vi "Filmetrics.vi"() -> ()   [LabVIEW 2018]
uses:
  <vilib>/Utility/file.llb/Write Delimited Spreadsheet (DBL).vi
  <vilib>/Utility/file.llb/Read Delimited Spreadsheet (DBL).vi
panel:
  in  "Accumulation times":sgl=1.0 min=1 step=1 format="%#_1g"
  in  "Substrate":string(combo)
  in  "Accumulation?":bool
  in  "Guessing Thickness(nm)3":string
  in  "Guessing Thickness(nm)2":string
  in  "Guessing Thickness(nm)1":string
  in  "Layer 3 Material":string(combo)
  in  "Layer 2 Material":string(combo)
  in  "Layer 1 Material":string(combo)
  in  "Calculate Thickness":bool
  out "Layers Ready":bool
  in  "Set layers":bool
  in  "Number of layers":sgl=1.0 min=1 max=3 step=1
  out "Raw Intensity Graph":T1(graph)
  out "Reflectance vs. Wavelength Graph":cluster{"all rows":dbl[], "all rows":dbl[]}[](graph)
  out "Display":string
  out "Scan Completed?":bool
  out "Counts":i32
  in  "Measurement":enum16{"Background", "Silicon", "Sample"}(ring)
  in  "Start Scan":bool
  in  "Stop Scan":bool
  in  "Integration Time [s] (0.001)":dbl=0.01 min=0.01
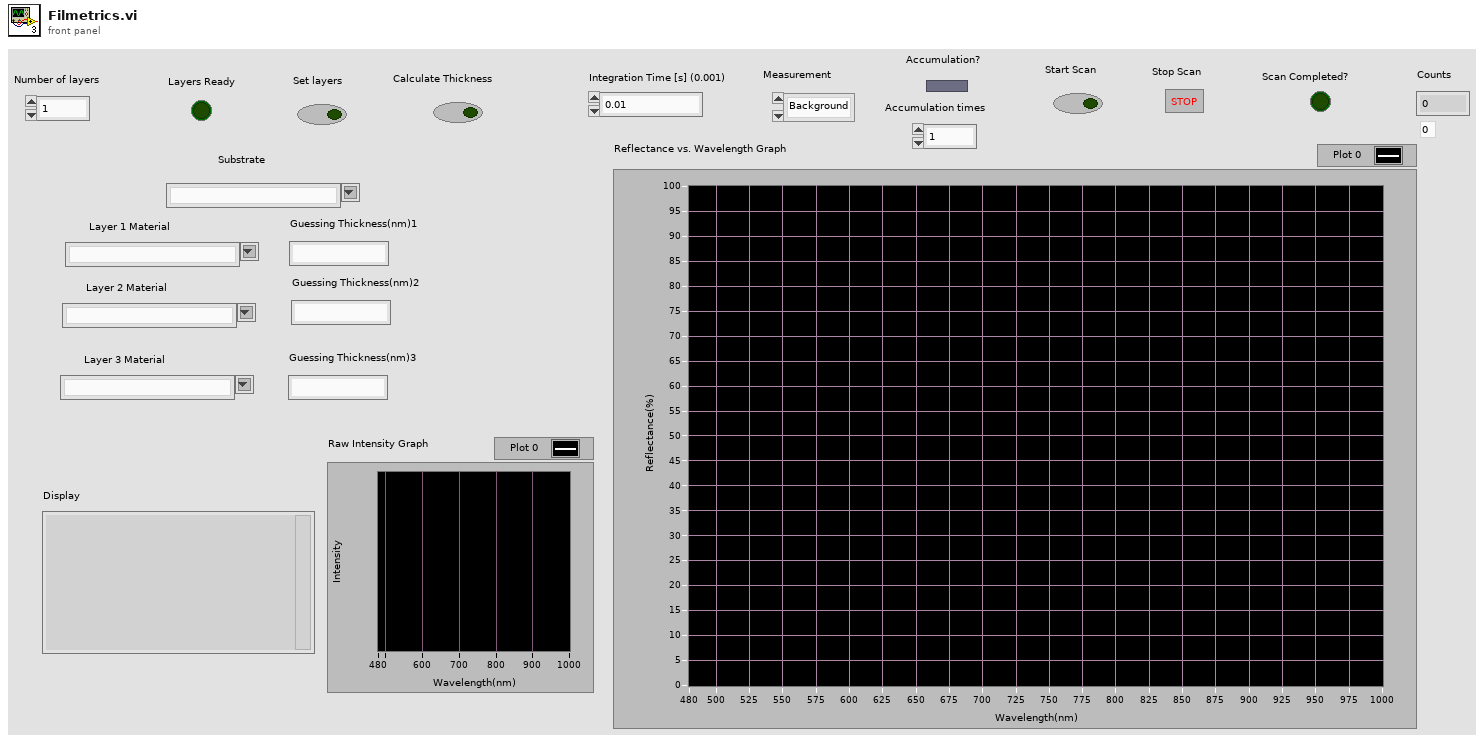
[diagram p1: front panel]
types:
  T1 = cluster{"Wavelength Data Array":dbl[], "Data":dbl[]}
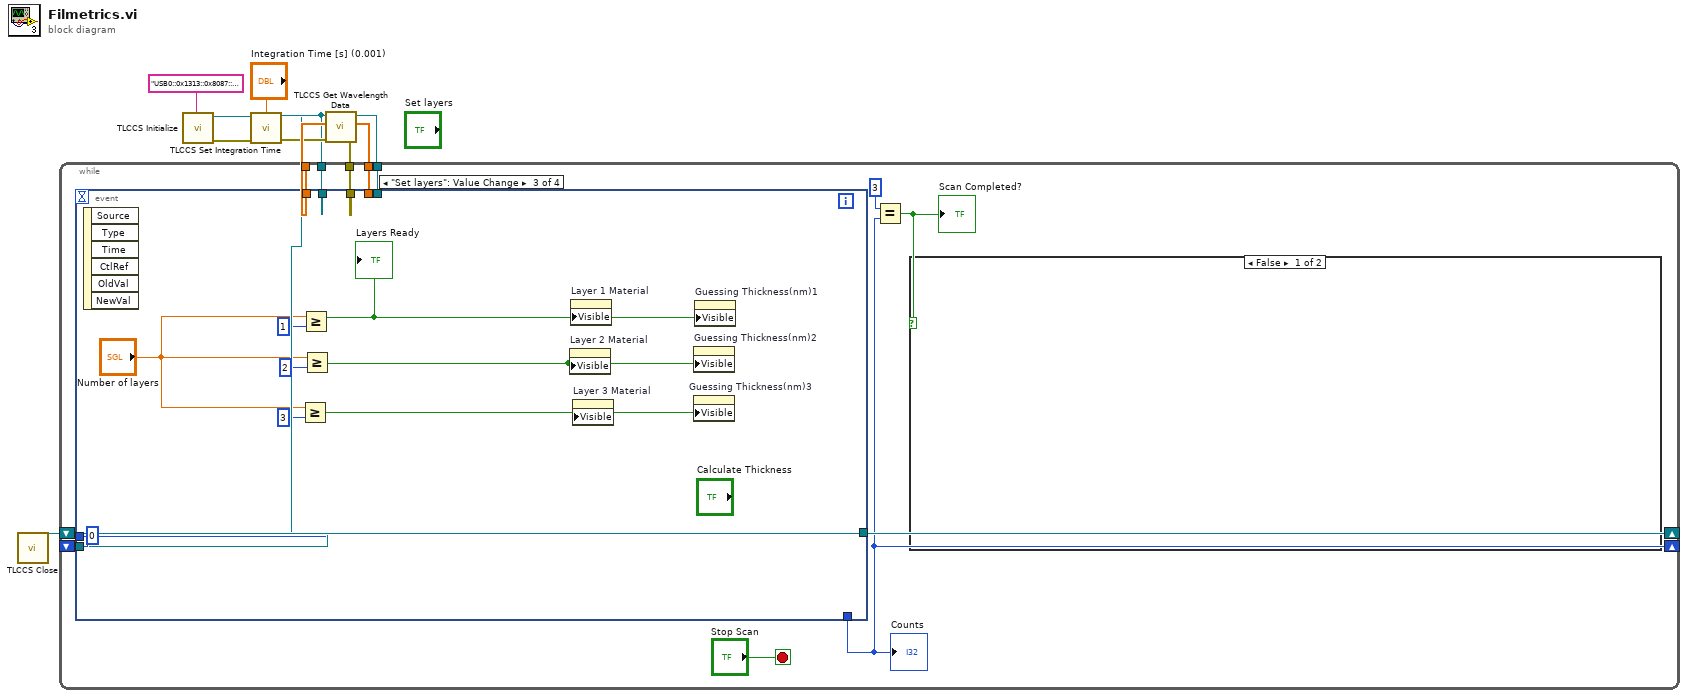
[diagram p0: block diagram]
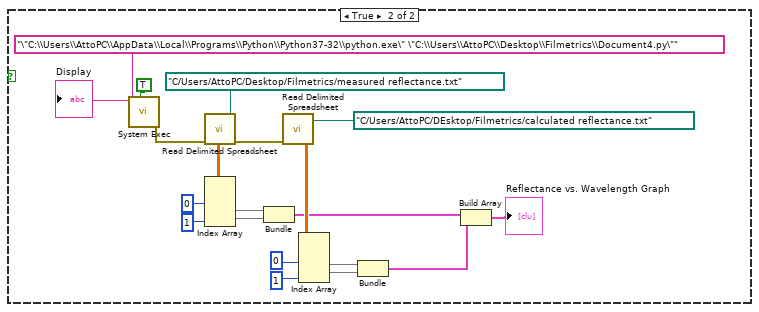
[diagram p2: hidden frame]
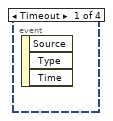
[diagram p3: hidden frame]
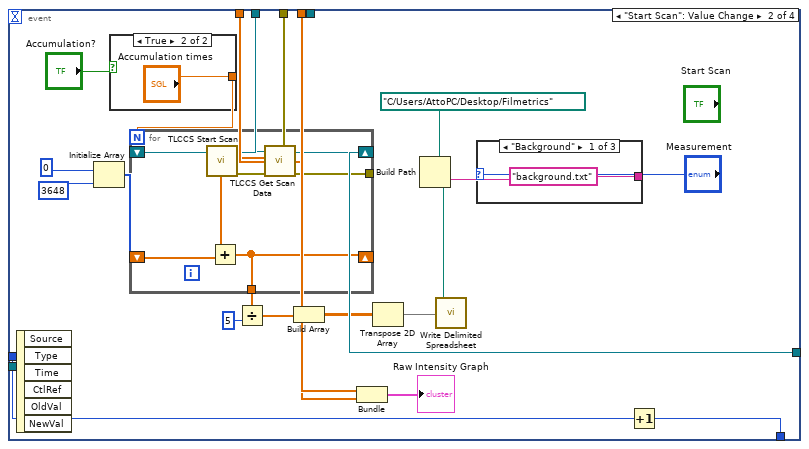
[diagram p4: hidden frame]
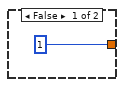
[diagram p5: hidden frame]
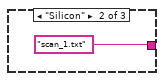
[diagram p6: hidden frame]
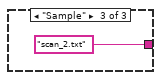
[diagram p7: hidden frame]
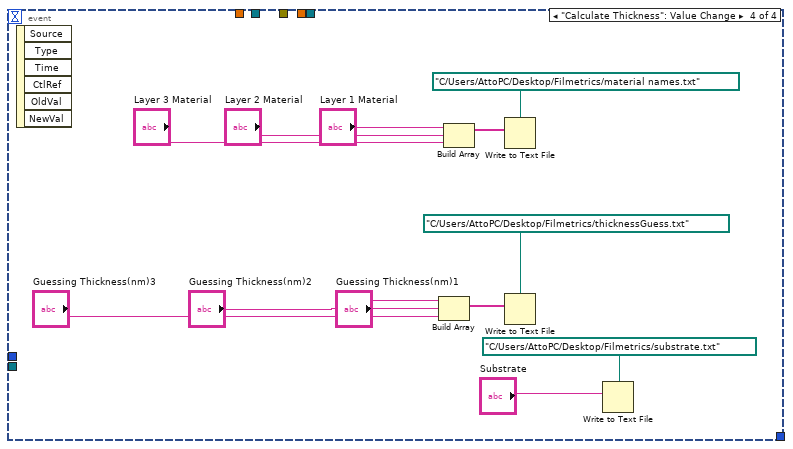
[diagram p8: hidden frame]
diagram:
  n1 = call <instrlib>:"TLCCS Initialize.vi"("resource name"="USB0::0x1313::0x8087::M00457586::RAW") -> ("error out"=w5:errorcluster, "instrument handle out"=w2:refnum<visa-resource-name>)  [unwired: 9 in]
  n2 = call <instrlib>:"TLCCS Set Integration Time.vi"("error in (no error)"=w5, "Integration Time [s] (0.001)"="Integration Time [s] (0.001)", "instrument handle"=w2) -> ("error out"=w4:errorcluster, "instrument handle out"=w9:refnum<visa-resource-name>)  [unwired: 7 in]
  n3 = call <instrlib>:"TLCCS Get Wavelength Data.vi"("error in (no error)"=w4, "instrument handle"=w9) -> ("error out"=w3:errorcluster, "Wavelength Data Array"=w6:dbl[], "instrument handle out"=w1:refnum<visa-resource-name>)  [unwired: 5 in, 2 out]
  n4 = while {
    tunnel: w6 -> [w15]
    shift-right: [w22] -> w10
    shift-left: w1 -> [w23]
    shift-right: [w12] -> _
    shift-left: 0 -> [w21]
    tunnel: w6 -> [w16]
    tunnel: w3 -> [w17]
    tunnel: w1 -> [w14]
    tunnel: w1 -> [w13]
    stop <- "Stop Scan" stop-if-true
    n5 = event shown="[2] \"Set layers\": Value Change" {
      selector: _ -> [_ _ _ _]
      dyn-events: _ -> [_ _ _ _]
      timeout: _ -> [_ _ _ _]
      tunnel: w23 -> [_ _ _ _]
      tunnel: [_ w65 _ _] -> w22
      tunnel: w21 -> [_ w59 _ _]
      tunnel: w17 -> [_ w53 _ _]
      tunnel: w16 -> [_ w62 _ _]
      tunnel: w15 -> [_ w60 _ _]
      tunnel: [_ w58 _ _] -> w12
      tunnel: w14 -> [_ w56 _ _]
      tunnel: w13 -> [_ _ _ _]
      event Timeout {
        n6 = event-data() -> ()  [unwired: 1 in, 3 out]
      }
      event "Start Scan": Value Change {
        n7 = event-data() -> ()  [unwired: 1 in, 6 out]
        n8 = Initialize Array(0, 3648) -> (w47:i32[])
        n9 = case shown="True" "Accumulation?" {
          tunnel: [1 "Accumulation times"] -> w50
          frame False {
          }
          frame True {
          }
        }
        n10 = for {
          N: w50 -> [_]
          tunnel: [w68] -> w46
          tunnel: w53 -> [w70]
          shift-right: [w73] -> w65
          shift-left: w56 -> [w72]
          shift-right: [w68] -> _
          shift-left: w47 -> [w66]
          n11 = call <instrlib>:"TLCCS Start Scan.vi"("error in (no error)"=w70, "instrument handle"=w72) -> ("error out"=w69:errorcluster, "instrument handle out"=w71:refnum<visa-resource-name>)  [unwired: 8 in]
          n12 = call <instrlib>:"TLCCS Get Scan Data.vi"("error in (no error)"=w69, "instrument handle"=w71) -> ("Data"=w67:dbl[], "instrument handle out"=w73:refnum<visa-resource-name>)  [unwired: 7 in, 1 out]
          n13 = Add(x=w67, y=w66) -> (x+y=w68:dbl[])
        }
        n14 = Divide(x=w46, y=5) -> (x/y=w44:dbl[])
        n15 = Build Array(w60, w44) -> (w64:dbl[][])
        n16 = Bundle("Wavelength Data Array"=w62, w44) -> (→"Raw Intensity Graph":cluster{"Wavelength Data Array":dbl[], dbl[]})  [unwired: 1 in]
        n17 = Transpose 2D Array(2D array=w64) -> (transposed array=w54:dbl[][])
        n18 = case shown="\"Background\"" "Measurement" {
          tunnel: ["background.txt" "scan_1.txt" "scan_2.txt"] -> w57
          frame "Background" {
          }
          frame "Silicon" {
          }
          frame "Sample" {
          }
        }
        n19 = Build Path(base path=path "C:/Users/AttoPC/Desktop/Filmetrics", name or relative path=w57) -> (appended path=w55:path)
        n20 = call-poly <vilib>:"Write Delimited Spreadsheet.vi"("file path (dialog if empty)"=w55, "2D data"=w54) -> ()  [unwired: 12 in, 2 out]
        n21 = Increment(x=w59) -> (x+1=w58:i32)
      }
      event "Set layers": Value Change {
        n22 = event-data() -> ()  [unwired: 1 in, 6 out]
        n23 = Greater Or Equal?(x="Number of layers", y=3) -> (x >= y?=w81:bool)
        n24 = Greater Or Equal?(x="Number of layers", y=1) -> (x >= y?=w80:bool)
        "Layers Ready" <- w80
        n25 = Greater Or Equal?(x="Number of layers", y=2) -> (x >= y?=w79:bool)
        n26 = property on="Layer 2 Material" class="CmbBox"("Visible"=w79) -> ()  [unwired: 2 in, 2 out]
        n27 = property on="Layer 1 Material" class="CmbBox"("Visible"=w80) -> ()  [unwired: 2 in, 2 out]
        n28 = property on="Layer 3 Material" class="CmbBox"("Visible"=w81) -> ()  [unwired: 2 in, 2 out]
        n29 = property on="Guessing Thickness(nm)2" class="Str"("Visible"=w79) -> ()  [unwired: 2 in, 2 out]
        n30 = property on="Guessing Thickness(nm)3" class="Str"("Visible"=w81) -> ()  [unwired: 2 in, 2 out]
        n31 = property on="Guessing Thickness(nm)1" class="Str"("Visible"=w80) -> ()  [unwired: 2 in, 2 out]
      }
      event "Calculate Thickness": Value Change {
        n32 = event-data() -> ()  [unwired: 1 in, 6 out]
        n33 = Build Array("Guessing Thickness(nm)1", "Guessing Thickness(nm)2", "Guessing Thickness(nm)3") -> (w88:string[])
        n34 = Build Array("Layer 1 Material", "Layer 2 Material", "Layer 3 Material") -> (w89:string[])
        n35 = Write to Text File(file (use dialog)=path "C:/Users/AttoPC/Desktop/Filmetrics/material names.txt", text=w89) -> ()  [unwired: 2 in, 3 out]
        n36 = Write to Text File(file (use dialog)=path "C:/Users/AttoPC/Desktop/Filmetrics/thicknessGuess.txt", text=w88) -> ()  [unwired: 2 in, 3 out]
        n37 = Write to Text File(file (use dialog)=path "C:/Users/AttoPC/Desktop/Filmetrics/substrate.txt", text="Substrate") -> ()  [unwired: 2 in, 3 out]
      }
    }
    "Counts" <- w12
    n38 = Equal?(x=3, y=w12) -> (x = y?=w18:bool)
    "Scan Completed?" <- w18
    n39 = case shown="False" w18 {
      frame False {
      }
      frame True {
        n40 = call <vilib>:"System Exec.vi"("wait until completion? (T)"=TRUE, "command line"="\"C:\\Users\\AttoPC\\AppData\\Local\\Programs\\Python\\Python37-32\\python.exe\" \"C:\\Users\\AttoPC\\Desktop\\Filmetrics\\Document4.py\"") -> ("error out"=w35:errorcluster, "standard output"=→"Display":string)  [unwired: 6 in, 2 out]
        n41 = call-poly <vilib>:"Read Delimited Spreadsheet.vi"("file path (dialog if empty)"=path "C:/Users/AttoPC/Desktop/Filmetrics/measured reflectance.txt", "error in (no error)"=w35) -> ("all rows"=w40:dbl[][], "error out"=w24:errorcluster)  [unwired: 8 in, 4 out]
        n42 = Index Array(array=w40, index (col) #1=0 ("disabled index (col)"), index (col) #2=1 ("index (col)")) -> (element #1=w37:dbl[], element #2=w36:dbl[])  [unwired: 2 in]
        n43 = Bundle("all rows"=w37, "all rows"=w36) -> (w27:cluster{"all rows":dbl[], "all rows":dbl[]})  [unwired: 1 in]
        n44 = call-poly <vilib>:"Read Delimited Spreadsheet.vi"("file path (dialog if empty)"=path "C:/Users/AttoPC/DEsktop/Filmetrics/calculated reflectance.txt", "error in (no error)"=w24) -> ("all rows"=w32:dbl[][])  [unwired: 8 in, 5 out]
        n45 = Index Array(array=w32, index (col) #1=0 ("disabled index (col)"), index (col) #2=1 ("index (col)")) -> (element #1=w29:dbl[], element #2=w28:dbl[])  [unwired: 2 in]
        n46 = Bundle("all rows"=w29, "all rows"=w28) -> (w26:cluster{"all rows":dbl[], "all rows":dbl[]})  [unwired: 1 in]
        n47 = Build Array(w27, w26) -> (→"Reflectance vs. Wavelength Graph":cluster{"all rows":dbl[], "all rows":dbl[]}[])
      }
    }
  }
  n48 = call <instrlib>:"TLCCS Close.vi"("instrument handle"=w10) -> ()  [unwired: 10 in, 1 out]
